vi "Initialise.vi"(8 "error in (no error)":errorcluster, 10 "Message in":refnum<class "InitialiseMessage.lvclass">, 11 "LineCCD in":refnum<class "LineCCD.lvclass">) -> (0 "error out":errorcluster, 3 "LineCCD out":refnum<class "LineCCD.lvclass">)   [LabVIEW 2012, in "LineCCD.lvclass"]
doc: "This method is called when an initialise message is received. It mainly initialises the RabbitMQ connectivity. \n\nOverride this method when your component needs special initialisation (e.g. of software or hardware resources). In that case, don't forget to call the parent for proper implementation. If your component owns subcomponents, they count as resources, so you have to initialise them by calling their own initialise functions"
uses:
  LineCCD.lvclass
  <vilib>/Distrio/Murmex/InitialiseMessage/InitialiseMessage.lvclass
  <vilib>/Distrio/Murmex/Murmex/Murmex.lvclass
  Fit ERF.ctl
  LineCCD.lvclass/LineCCD.ctl
  <instrlib>/ALPHALAS CCD S Series/ALPHALAS CCD S Series.lvlib
panel:
  # "This method is called when the INTIALISE\ntrigger is sent. \n\nOverride this method when your component needs to\nrespond to this trigger. \n\nCall parent for proper implementation"
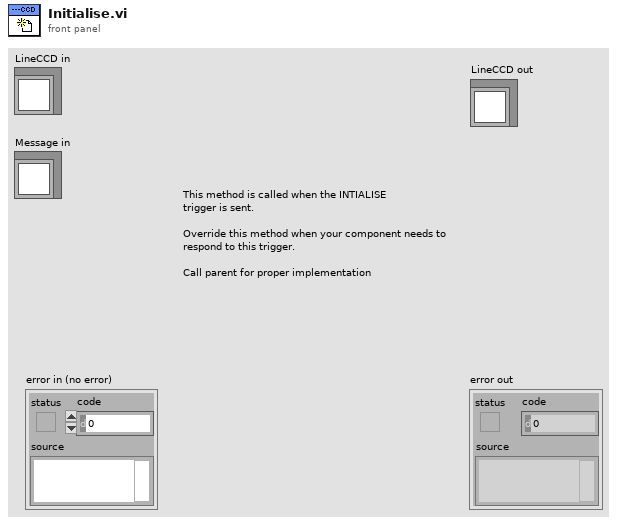
[diagram p1: front panel]
types:
  T1 = typedef "LineCCD.lvclass/Fit ERF.ctl" = enum16{"Default", "derivative 4x", "Fit ERF", "Fit ERF x4"}
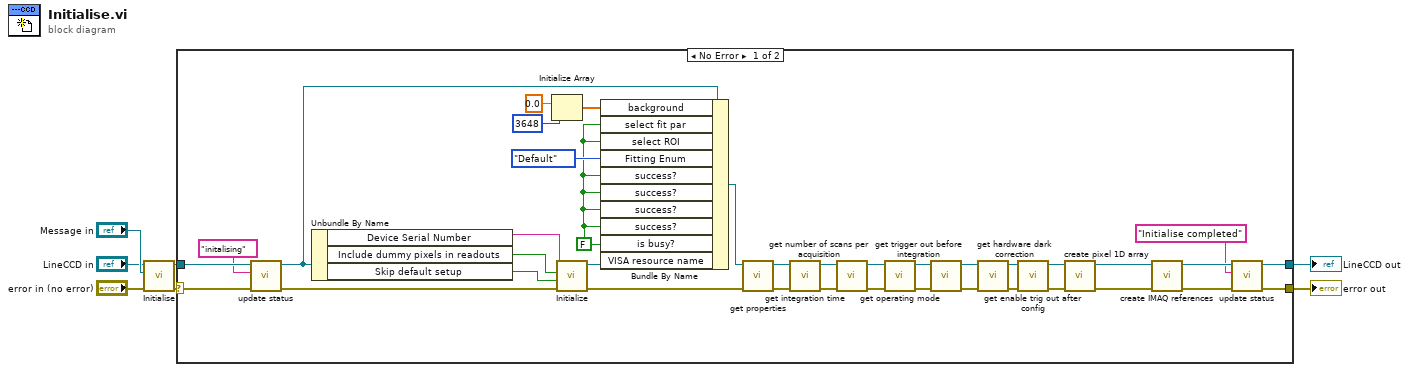
[diagram p0: block diagram]
diagram:
  n1 = call-parent "Initialise.vi"("error in (no error)"="error in (no error)", "Message in"="Message in", "Murmex in"="LineCCD in") -> ("error out"=w4:errorcluster, "Murmex out"=w3:refnum<class "LineCCD.lvclass">)  [unwired: 7 in]
  n2 = case shown="No Error" w4 {
    selector: w4 -> [w22 w45]
    tunnel: w3 -> [w21 w46]
    tunnel: [w14 w46] -> w2
    tunnel: [w16 w45] -> w1
    frame No Error {
      w23 = FALSE ("runtime.is busy?")
      n3 = call-dynamic "update status.vi"("error in (no error)"=w22, "String In"="initalising", "LineCCD in"=w21) -> ("error out"=w19:errorcluster, "LineCCD out"=w20:refnum<class "LineCCD.lvclass">)  [unwired: 7 in]
      n4 = Unbundle By Name(w20) -> ("Device Serial Number"=w44:string, "Include dummy pixels in readouts"=w27:bool, "Skip default setup"=w43:bool)
      n5 = Initialize Array(0.0 ("element"), 3648 ("dimension size")) -> (w10:dbl[])
      n6 = call <instrlib>:"Initialize.vi"("error in (no error)"=w19, "Skip Default Setup (False)"=w43, "Include Dummy Pixels in Readouts (False)"=w27, "Device Serial Number"=w44) -> ("error out"=w40:errorcluster, "VISA resource name out"=w42:refnum<visa-resource-name>)  [unwired: 6 in]
      n7 = Bundle By Name(cluster=w20, "background"=w10, "select fit par"=w23, "select ROI"=w23, "Fitting Enum"=Fit_ERF."Default" ("runtime.Fitting.Fitting Enum"), "success?"=w23, "success?"=w23, "success?"=w23, "success?"=w23, "is busy?"=w23, "VISA resource name"=w42) -> (w41:refnum<class "LineCCD.lvclass">)
      n8 = call-dynamic "get properties.vi"("error in (no error)"=w40, "LineCCD in"=w41) -> ("error out"=w39:errorcluster, "LineCCD out"=w33:refnum<class "LineCCD.lvclass">)  [unwired: 8 in]
      n9 = call-dynamic "get integration time.vi"("error in (no error)"=w39, "LineCCD in"=w33) -> ("error out"=w38:errorcluster, "LineCCD out"=w32:refnum<class "LineCCD.lvclass">)  [unwired: 7 in, 1 out]
      n10 = call-dynamic "get number of scans per acquisition.vi"("error in (no error)"=w38, "LineCCD in"=w32) -> ("error out"=w37:errorcluster, "LineCCD out"=w31:refnum<class "LineCCD.lvclass">)  [unwired: 8 in]
      n11 = call-dynamic "get operating mode.vi"("error in (no error)"=w37, "LineCCD in"=w31) -> ("error out"=w36:errorcluster, "LineCCD out"=w30:refnum<class "LineCCD.lvclass">)  [unwired: 8 in]
      n12 = call-dynamic "get trigger out before integration.vi"("error in (no error)"=w36, "LineCCD in"=w30) -> ("error out"=w35:errorcluster, "LineCCD out"=w29:refnum<class "LineCCD.lvclass">)  [unwired: 8 in]
      n13 = call-dynamic "get hardware dark correction.vi"("error in (no error)"=w35, "LineCCD in"=w29) -> ("error out"=w34:errorcluster, "LineCCD out"=w28:refnum<class "LineCCD.lvclass">)  [unwired: 8 in]
      n14 = call-dynamic "get enable trig out after config.vi"("error in (no error)"=w34, "LineCCD in"=w28) -> ("error out"=w26:errorcluster, "LineCCD out"=w25:refnum<class "LineCCD.lvclass">)  [unwired: 8 in]
      n15 = call-dynamic "create pixel 1D array.vi"("error in (no error)"=w26, "LineCCD in"=w25) -> ("error out"=w8:errorcluster, "LineCCD out"=w9:refnum<class "LineCCD.lvclass">)  [unwired: 8 in]
      n16 = call-dynamic "create IMAQ references.vi"("error in (no error)"=w8, "LineCCD in"=w9) -> ("error out"=w17:errorcluster, "LineCCD out"=w15:refnum<class "LineCCD.lvclass">)  [unwired: 8 in]
      n17 = call-dynamic "update status.vi"("error in (no error)"=w17, "String In"="Initialise completed", "LineCCD in"=w15) -> ("error out"=w16:errorcluster, "LineCCD out"=w14:refnum<class "LineCCD.lvclass">)  [unwired: 7 in]
    }
    frame Error {
    }
  }
  "error out" <- w1
  "LineCCD out" <- w2
